vi "reponsegetport.vi"(8 "error in (no error)":errorcluster, 11 "NXP in":refnum<class "NXP.lvclass">) -> (0 "error out":errorcluster, 2 "String":string, 3 "NXP out":refnum<class "NXP.lvclass">)   [LabVIEW 2019, in "NXP.lvclass"]
uses:
  NXP.lvclass
  NXP.lvclass/NXP.ctl
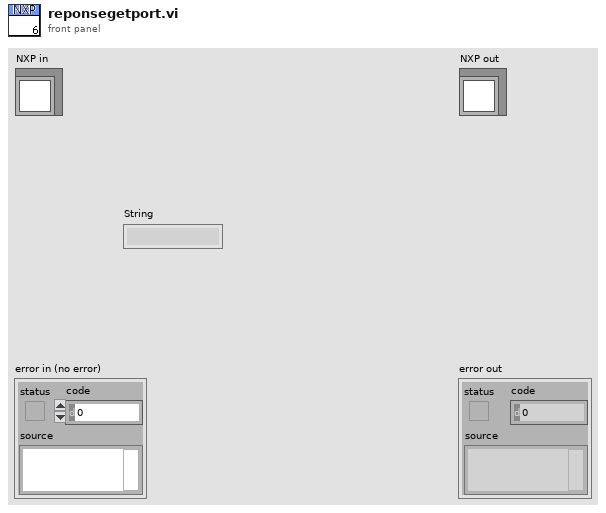
[diagram p1: front panel]
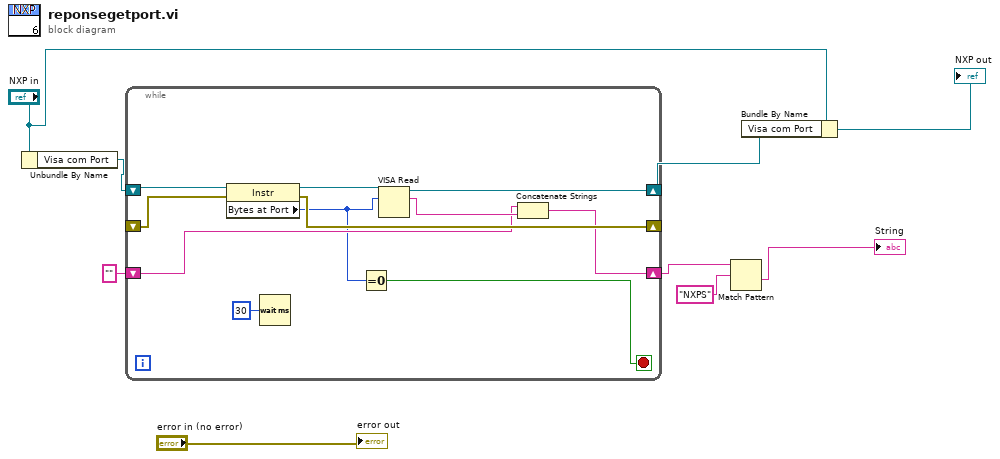
[diagram p0: block diagram]
diagram:
  n1 = Unbundle By Name("NXP in") -> ("Visa com Port"=w9:refnum<visa-resource-name>)
  n2 = while {
    shift-right: [w17] -> w5
    shift-left: w9 -> [w20]
    shift-right: [w16] -> _
    shift-left: _ -> [w15]
    shift-right: [w12] -> w4
    shift-left: "" -> [w13]
    stop <- w10 stop-if-true
    n3 = property class="Instr"(reference=w20, error in=w15) -> (reference out=w18:refnum<visa-resource-name>, error out=w16:errorcluster, "Bytes at Port"=w11:u32)
    n4 = Wait (ms)(milliseconds to wait=u32 30) -> ()  [unwired: 1 out]
    n5 = Equal To 0?(x=w11) -> (x = 0?=w10:bool)
    n6 = VISA Read(VISA resource name=w18, byte count=w11) -> (VISA resource name out=w17:refnum<visa-resource-name>, read buffer=w14:string)  [unwired: 1 in, 2 out]
    n7 = Concatenate Strings(w13, w14) -> (w12:string)
  }
  n8 = Match Pattern(string=w4, regular expression="NXPS") -> (after substring=→"String":string)  [unwired: 1 in, 3 out]
  n9 = Bundle By Name(cluster="NXP in", "Visa com Port"=w5) -> (→"NXP out":refnum<class "NXP.lvclass">)
  "error out" <- "error in (no error)"
